vi "Rx Construct.vi"(6 "received messages":T1[](array[typedef]) {"Timestamp Channel Handle" format="%.0x"; "Message Section Handle" format="%.0x"; "Parameter Channel Handles" format="%.0x"}, 8 "error in":errorcluster, 10 "biu configuration":T5, 11 "id":string) -> (0 "error out":errorcluster, 3 "rx execution unit":refnum<class "Rx Execution Unit.lvclass">)   [LabVIEW 2020, in "AIM MIL-STD-1553 Engine.lvlib" / "Implementation.lvlib" / "Rx Execution Unit.lvclass"]
uses:
  Rx Execution Unit.lvclass
  C:/dev/git/niveristand-aim-milStd1553-custom-device/Source/Custom Device Support/Engine/Implementation/Execution Unit/Execution Unit.lvclass
  Shared/BIU Configuration.ctl
  Shared/Address.ctl
  Shared/Major Frame Definition.ctl
  Shared/Minor Frame Definition.ctl
  Shared/Message Definition.ctl
  Shared/Message Type.ctl
  Shared/Terminal Endpoint.ctl
  Shared/Parameter Definition.ctl
  Custom Device/Compiled Message.ctl
  <vilib>/NI VeriStand/Custom Device API/Custom Device Item Ref.ctl
  Shared/Direction.ctl
  Rx Execution Unit.lvclass/Rx Execution Unit.ctl
  Execution Unit/Execution Unit.lvclass
  <vilib>/NI VeriStand/Custom Device API/Custom Device API.lvlib
  Custom Device/Custom Device.lvlib
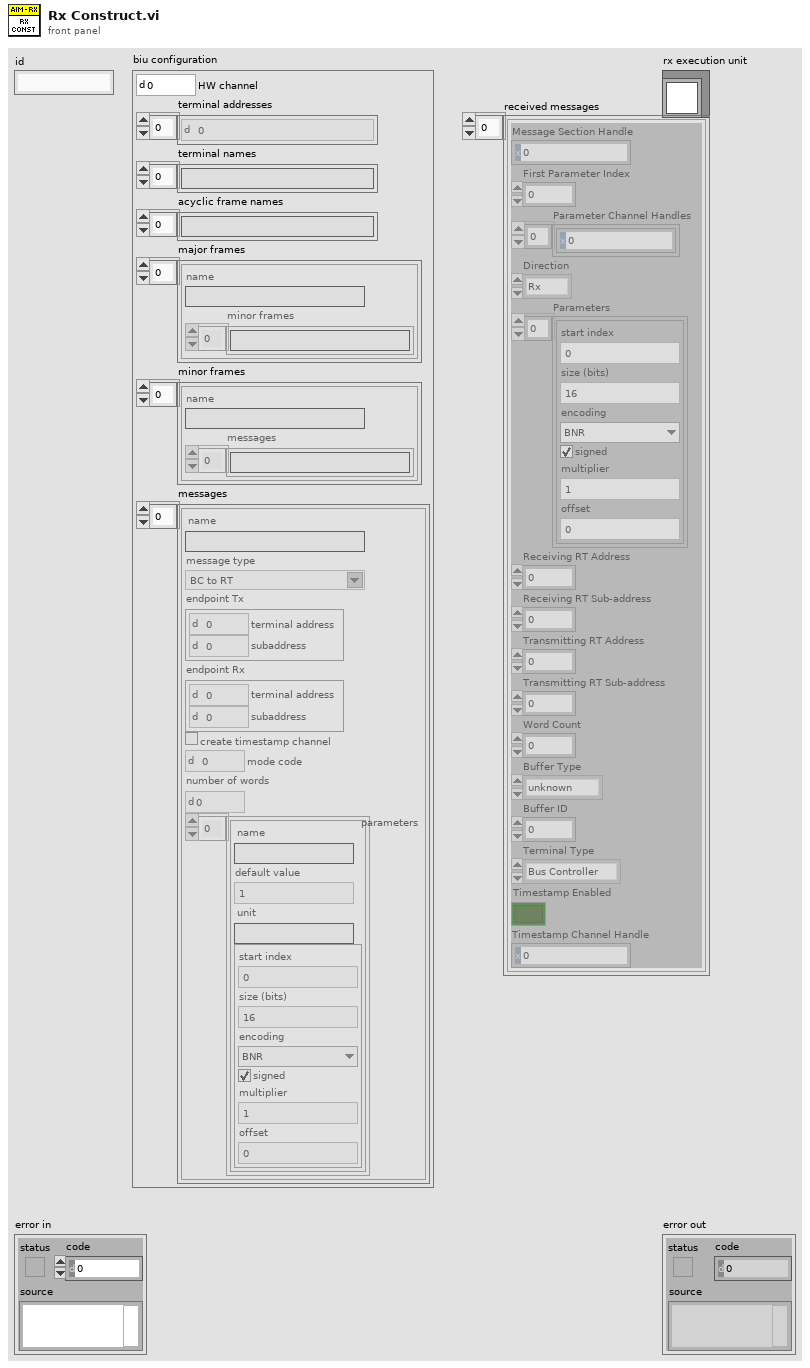
[diagram p1: front panel]
types:
  T1 = typedef "AIM MIL-STD-1553 Engine.lvlib/Custom Device.lvlib/Compiled Message.ctl" = cluster{"Message Section Handle":T2, "First Parameter Index":i32, "Parameter Channel Handles":T2[], "Direction":T3, "Parameters":T4[], "Receiving RT Address":u8, "Receiving RT Sub-address":u8, "Transmitting RT Address":u8, "Transmitting RT Sub-address":u8, "Word Count":u8, "Buffer Type":enum16{"unknown", "BC Message Buffer", "RT Message Buffer"}, "Buffer ID":u16, "Terminal Type":enum16{"Bus Controller", "Remote Terminal"}, "Timestamp Enabled":bool, "Timestamp Channel Handle":T2}
  T2 = typedef "Custom Device API.lvlib/Custom Device Item Ref.ctl" = u64
  T3 = typedef "Direction.ctl" = enum16{"Rx", "Tx"}
  T4 = typedef "Parameter Definition.ctl" = cluster{"start index":i32, "size (bits)":i32, "encoding":enum16{"BNR", "BCD", "Discrete"}, "signed":bool, "multiplier":dbl, "offset":dbl}
  T5 = typedef "BIU Configuration.ctl" = cluster{"HW channel":u16, "terminal addresses":T6[], "terminal names":string[], "acyclic frame names":string[], "major frames":T7[], "minor frames":T8[], "messages":T9[]}
  T6 = typedef "Address.ctl" = u16
  T7 = typedef "Major Frame Definition.ctl" = cluster{"name":string, "minor frames":string[]}
  T8 = typedef "Minor Frame Definition.ctl" = cluster{"name":string, "messages":string[]}
  T9 = typedef "Message Definition.ctl" = cluster{"name":string, "message type":T10, "endpoint Tx":T11, "endpoint Rx":T11, "create timestamp channel":bool, "mode code":u16, "number of words":u16, "parameters":cluster{"name":string, "default value":dbl, "unit":string, "parameter definition":T4}[]}
  T10 = typedef "Message Type.ctl" = string
  T11 = typedef "Terminal Endpoint.ctl" = cluster{"terminal address":T6, "subaddress":T6}
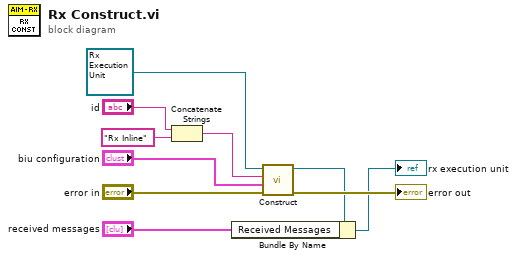
[diagram p0: block diagram]
diagram:
  n1 = Concatenate Strings("id", "Rx Inline" ("id")) -> (w1:string)
  n2 = call "Construct.vi"("error in"="error in", "biu configuration"="biu configuration", "id"=w1, "execution unit"=refnum<class "Rx Execution Unit.lvclass"> refnum ("Communication Bus Template Interfaces:Implementation.lvlib:Rx Execution Unit.lvclass")) -> ("error out"=→"error out":errorcluster, "execution unit out"=w6:refnum<class "Rx Execution Unit.lvclass">)  [unwired: 6 in]
  n3 = Bundle By Name(cluster=w6, "Received Messages"="received messages") -> (→"rx execution unit":refnum<class "Rx Execution Unit.lvclass">)
